vi "GetVel.vi"(10 "Position":dbl[](array[numeric]), 11 "FrameNum":dbl) -> (3 "Velocity":dbl[](array[numeric]))   [LabVIEW 2017]
uses:
  <vilib>/Analysis/3filter.llb/Filter Passband Type.ctl
  <vilib>/ptbypt/NI_PtbyPt.lvlib
  <vilib>/Analysis/NI_AALBase.lvlib
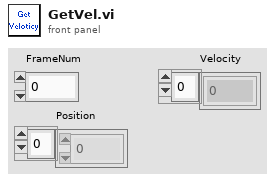
[diagram p1: front panel]
types:
  T1 = typedef "NI_AALBase.lvlib/Filter Passband Type.ctl" = enum32{"Lowpass", "Highpass", "Bandpass", "Bandstop"}
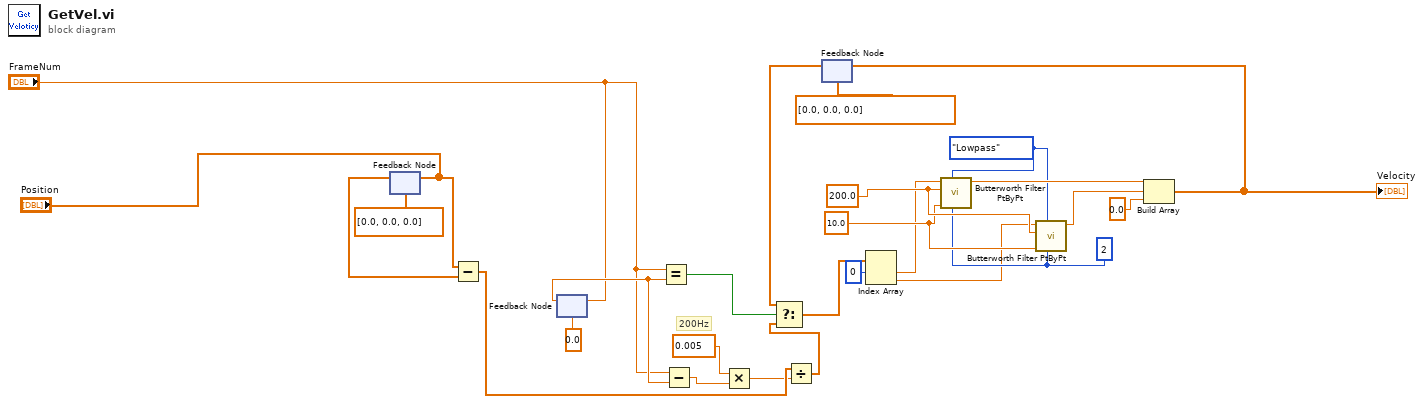
[diagram p0: block diagram]
diagram:
  w22 = 10.0
  w23 = 200.0
  w18 = 2 ("order")
  w15 = Filter_Passband_Type."Lowpass" ("filter type")
  # "200Hz"
  n1 = feedback #1(dbl[] [0.0, 0.0, 0.0]) -> (w12:dbl[])
  n2 = feedback-in #1("Position") -> ()
  n3 = Subtract(x="Position", y=w12) -> (x-y=w11:dbl[])
  n4 = feedback #2(0.0 ("FrameNum")) -> (w4:dbl)
  n5 = feedback-in #2("FrameNum") -> ()
  n6 = Equal?(x="FrameNum", y=w4) -> (x = y?=w2:bool)
  n7 = Subtract(x="FrameNum", y=w4) -> (x-y=w6:dbl)
  n8 = Multiply(x=0.005, y=w6) -> (x*y=w7:dbl)
  n9 = Divide(x=w11, y=w7) -> (x/y=w8:dbl[])
  n10 = feedback #3(dbl[] [0.0, 0.0, 0.0]) -> (w25:dbl[])
  n11 = Select(t=w25, s=w2, f=w8) -> (s? t:f=w13:dbl[])
  n12 = Index Array(array=w13, index #1=0 ("index")) -> (element #1=w16:dbl, element #2=w17:dbl)  [unwired: 1 in]
  n13 = call <vilib>:"Butterworth Filter PtByPt.vi"("order"=w18, "filter type"=w15, "low cutoff freq: fl"=w22, "sampling freq: fs"=w23, "x"=w16) -> ("Filtered x"=w19:dbl)  [unwired: 4 in, 1 out]
  n14 = call <vilib>:"Butterworth Filter PtByPt.vi"("order"=w18, "filter type"=w15, "low cutoff freq: fl"=w22, "sampling freq: fs"=w23, "x"=w17) -> ("Filtered x"=w20:dbl)  [unwired: 4 in, 1 out]
  n15 = Build Array(w19, w20, 0.0) -> (w24:dbl[])
  "Velocity" <- w24
  n16 = feedback-in #3(w24) -> ()
